vi "FTW-Endpoint-TCP-Request-Worker-Start.vi"(0 "FTW-Endpoint-TCP In":refnum<class "FTW-Endpoint-TCP.lvclass">, 5 "Endpoint Address":string, 11 "error in":errorcluster) -> (4 "FTW-Endpoint-TCP Out":refnum<class "FTW-Endpoint-TCP.lvclass">, 15 "error out":errorcluster)   [LabVIEW 2015, in "FTW-Endpoint-TCP.lvclass"]
uses:
  FTW-Endpoint-TCP.lvclass
  FTW-Endpoint-TCP.lvclass/FTW-Endpoint-TCP.ctl
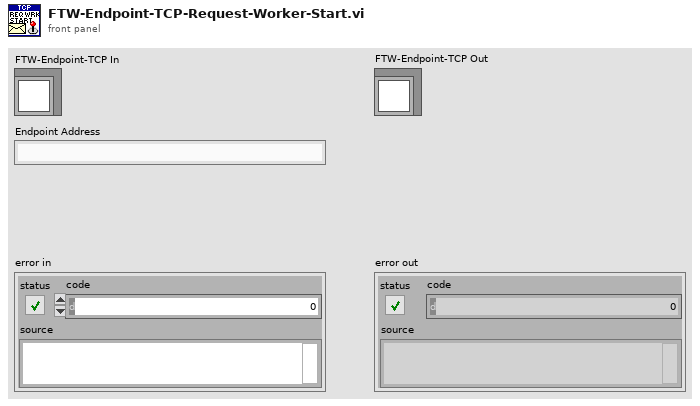
[diagram p1: front panel]
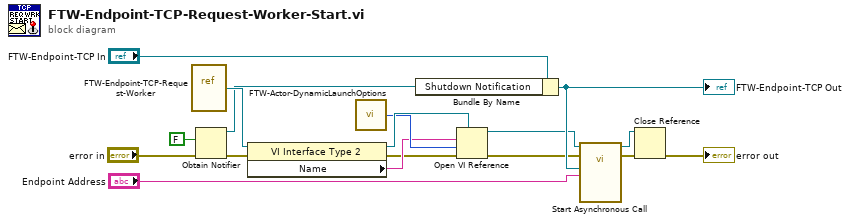
[diagram p0: block diagram]
diagram:
  n1 = vi-ref "FTW-Endpoint-TCP-Request-Worker.vi"() -> (w4:refnum<vi>)
  n2 = Obtain Notifier(notification data type=FALSE, error in (no error)="error in") -> (notifier out=w2:refnum<notifier>, error out=w1:errorcluster)  [unwired: 2 in, 1 out]
  n3 = property class="VI Interface Type 2"(reference=w4, error in=w1) -> (reference out=w8:refnum<vi>, error out=w5:errorcluster, "Name"=w6:string)
  n4 = call "FTW-Actor-DynamicLaunchOptions.vi"() -> ("Open VI Ref Options"=w7:i32)
  n5 = Bundle By Name(cluster="FTW-Endpoint-TCP In", "Shutdown Notification"=w2) -> (w15:refnum<class "FTW-Endpoint-TCP.lvclass">)
  "FTW-Endpoint-TCP Out" <- w15
  n6 = Open VI Reference(type specifier VI Refnum (for type only)=w8, vi path=w6, options=w7, error in (no error)=w5) -> (vi reference=w10:refnum<vi>, error out=w12:errorcluster)  [unwired: 2 in]
  n7 = call-by-ref "Start Asynchronous Call"(reference=w10, error in=w12, "TCP Endpoint"=w15, "Address"="Endpoint Address") -> (reference out=w11:refnum<vi>, error out=w9:errorcluster)  [unwired: 14 in]
  n8 = Close Reference(reference=w11, error in (no error)=w9) -> (error out=→"error out":errorcluster)
